vi "OAT Coerce Time Range.vi"(6 "scaled signal [EU] in":waveform(dbl), 7 "RPM range in":T1 {"Increment" format="%.2f"; "Maximum" format="%.2f"; "Minimum" format="%.2f"}) -> (2 "total rpm":i32, 3 "RPM range out":T1 {"Increment" format="%.2f"; "Maximum" format="%.2f"; "Minimum" format="%.2f"})   [LabVIEW 2017]
panel:
  # "Coerce Time Range"
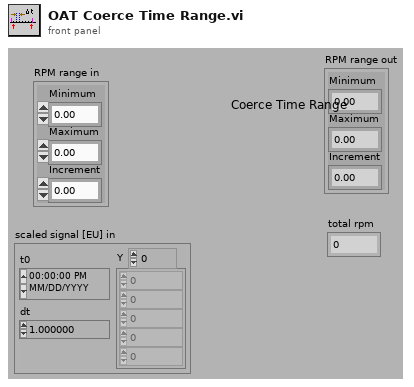
[diagram p1: front panel]
types:
  T1 = cluster{"Minimum":dbl, "Maximum":dbl, "Increment":dbl}
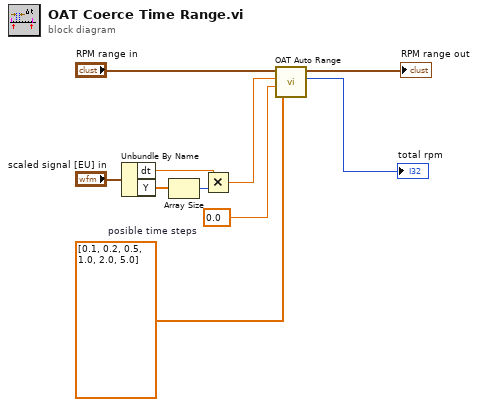
[diagram p0: block diagram]
diagram:
  w7 = dbl[] [0.1, 0.2, 0.5, 1.0, 2.0, 5.0]  # posible time steps
  n1 = Unbundle By Name("scaled signal [EU] in") -> ("dt"=w3:dbl, "Y"=w5:dbl[])
  n2 = Array Size(array=w5) -> (size(s)=w4:i32)
  n3 = Multiply(x=w3, y=w4) -> (x*y=w2:dbl)
  n4 = call <vilib>:"OAT Auto Range.vi"("posible increament"=w7, "lower limit"=0.0, "upper limit"=w2, "range in"="RPM range in") -> ("total step"=→"total rpm":i32, "range out"=→"RPM range out":T1)  [unwired: 6 in]
